vi "Sanitise Filename.vi"(8 "error in":errorcluster, 11 "input filename":string) -> (0 "error out":errorcluster, 3 "output filename":string)   [LabVIEW 2017]
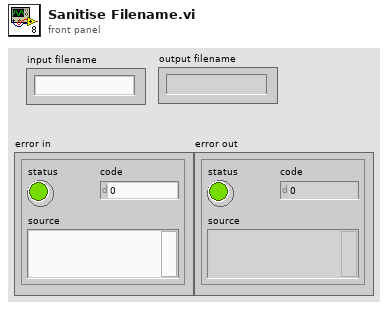
[diagram p1: front panel]
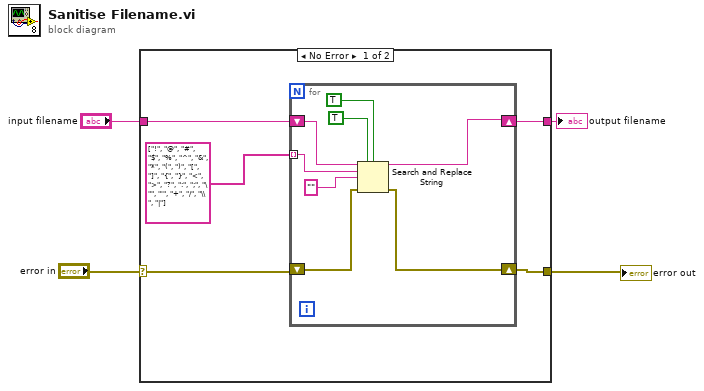
[diagram p0: block diagram]
diagram:
  n1 = case shown="No Error" "error in" {
    selector: "error in" -> [w6 w18]
    tunnel: "input filename" -> [w8 _]
    tunnel: [w7 _] -> w3
    tunnel: [w5 w18] -> w1
    frame No Error {
      n2 = for {
        tunnel: string[] ["!", "@", "#", "$", "%", "^", "&", "*", "(", ")", "[", "]", "{", "}", "<", ">", "?", ":", ";", "\"", "'", "+", "/", "\\", "|"] -> [w16] mode=indexing
        shift-right: [w12] -> w7
        shift-left: w8 -> [w17]
        shift-right: [w10] -> w5
        shift-left: w6 -> [w11]
        n3 = Search and Replace String(replace all?=TRUE ("replace all? (F)"), case sensitive?=TRUE ("ignore case? (F)"), input string=w17, search string=w16, replace string="" ("replace string (\"\")"), error in=w11) -> (result string=w12:string, error out=w10:errorcluster)  [unwired: 2 in, 2 out]
      }
    }
    frame Error {
    }
  }
  "error out" <- w1
  "output filename" <- w3
